vi "Replace Subset Array.vi"(2 "error in (no error)":errorcluster, 3 "new element/subarray":refnum<class "Generic Plugin.lvclass">[](array[class]), 4 "index":i32, 5 "Controller Array in":refnum<class "Controller Array.lvclass">) -> (0 "error out":errorcluster, 1 "Controller Array out":refnum<class "Controller Array.lvclass">)   [LabVIEW 2020, in "Controller Array.lvclass"]
uses:
  Controller Array.lvclass
  Controller/Generic Plugin.lvclass
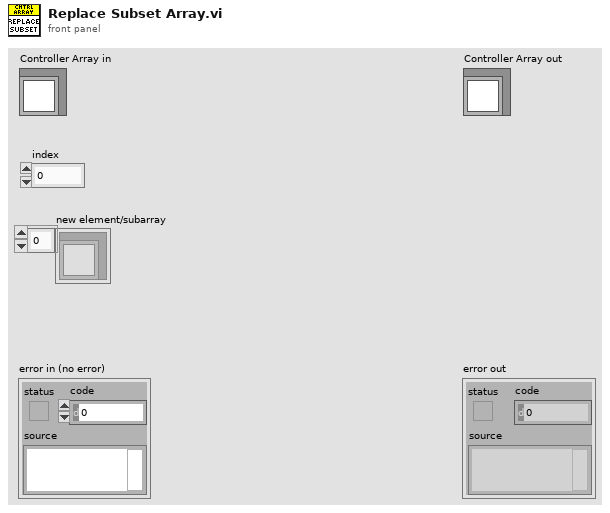
[diagram p1: front panel]
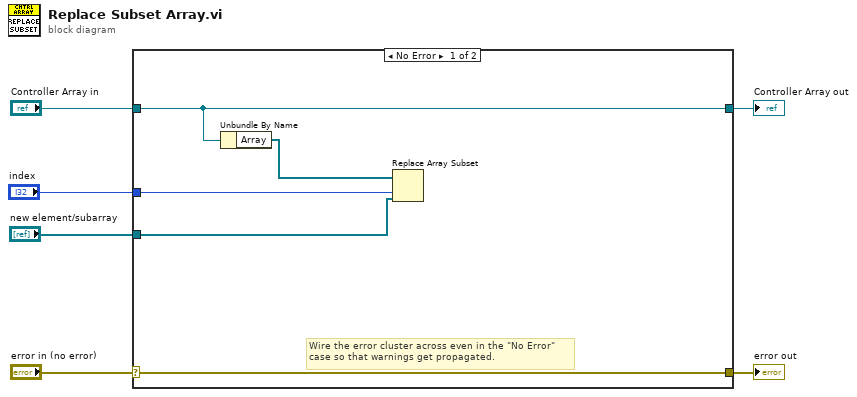
[diagram p0: block diagram]
diagram:
  n1 = case shown="No Error" "error in (no error)" {
    selector: "error in (no error)" -> [w11 w13]
    tunnel: [w11 w13] -> w5
    tunnel: [w10 w12] -> w3
    tunnel: "Controller Array in" -> [w10 w12]
    tunnel: "index" -> [w8 _]
    tunnel: "new element/subarray" -> [w7 _]
    frame No Error {
      # "Wire the error cluster across even in the \"No Error\"\ncase so that warnings get propagated."
      n2 = Unbundle By Name(w10) -> ("Array"=w9:refnum<class "Generic Plugin.lvclass">[])
      n3 = Replace Array Subset(array=w9, new element=w7, index=w8) -> ()  [unwired: 1 out]
    }
    frame Error {
    }
  }
  "error out" <- w5
  "Controller Array out" <- w3
